vi "SendToCaller.vi"(8 "error in (no error)":errorcluster, 9 "Data":variant, 10 "Command":T1, 11 "JQMHStartup in":refnum<class "RQMHStartup.lvclass">) -> (0 "error out":errorcluster, 3 "JQMHStartup out":refnum<class "RQMHStartup.lvclass">)   [LabVIEW 2024, in "RQMHStartup.lvclass"]
uses:
  RQMHStartup.lvclass
  Command.ctl
  Message.ctl
  RQMHStartup.lvclass/RQMHStartup.ctl
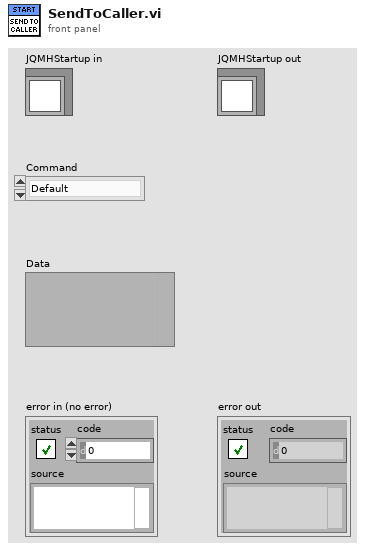
[diagram p1: front panel]
types:
  T1 = typedef "RQMHStartup.lvclass/Command.ctl" = enum16{"Default", "No Override", "Error", "ACK Created", "ACK Mod Reg", "ACK Caller Reg"}
  T2 = typedef "RQMHStartup.lvclass/Message.ctl" = cluster{"Command":T1, "Data":variant}
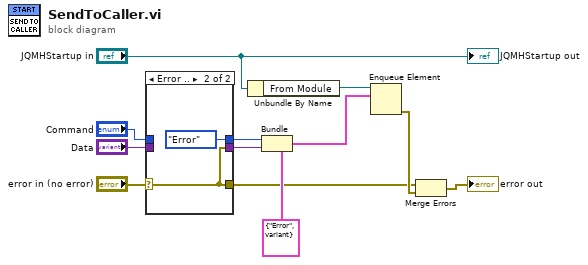
[diagram p0: block diagram]
diagram:
  n1 = case shown="Error .." "error in (no error)" {
    selector: "error in (no error)" -> [w13 w16]
    tunnel: [w15 Command."Error" ("Command")] -> w6
    tunnel: "Command" -> [w15 _]
    tunnel: "Data" -> [w14 _]
    tunnel: [w14 w16] -> w3
    tunnel: [w13 w16] -> w1
    frame No Error {
    }
    frame Error {
    }
  }
  n2 = Unbundle By Name("JQMHStartup in") -> ("From Module"=w10:refnum<queue>)
  n3 = Bundle(cluster=T2 {"Command"=enum."Error", "Data"=variant} ("element"), "Command"=w6, "Data"=w3) -> (w8:T2)
  n4 = Enqueue Element(queue=w10, element=w8) -> (error out=w12:errorcluster)  [unwired: 2 in, 2 out]
  n5 = Merge Errors(w1, w12) -> (→"error out":errorcluster)
  "JQMHStartup out" <- "JQMHStartup in"
